vi "CompileParseRFPulse.vi"(0 "String":string) -> (2 "Array":variant[](array[variant]))   [LabVIEW 2019]
panel:
  out "output cluster":T1
  in  "Channel cluster":T2(array[cluster])
  in  "Timing cluster":T3
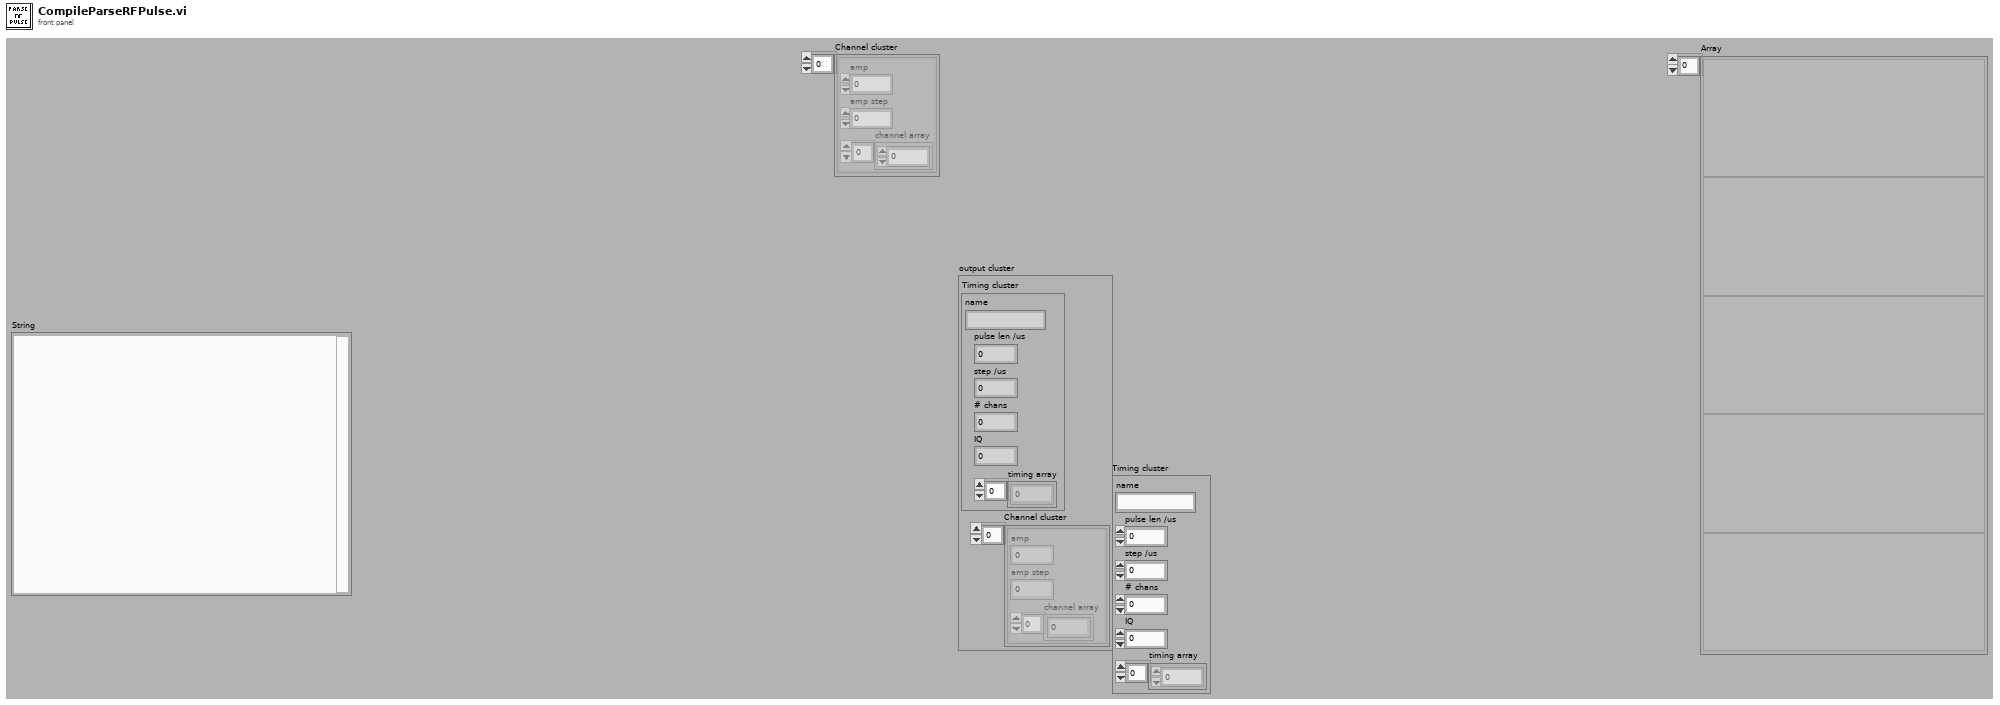
[diagram p1: front panel]
types:
  T1 = cluster{"Timing cluster":cluster{"name":string, "pulse len /us":dbl, "step /us":dbl, "# chans":i32, "IQ":i32, "timing array":dbl[]}, "Channel cluster":cluster{"amp":dbl, "amp step":dbl, "channel array":dbl[]}[]}
  T2 = cluster{"amp":dbl, "amp step":dbl, "channel array":dbl[]}[]
  T3 = cluster{"name":string, "pulse len /us":dbl, "step /us":dbl, "# chans":i32, "IQ":i32, "timing array":dbl[]}
  T4 = cluster{"Timing cluster 2":cluster{"name":string, "pulse len /us":dbl, "step /us":dbl, "# chans":i32, "IQ":i32, "timing array":dbl[]}, "Channel cluster 2":cluster{"amp":dbl, "amp step":dbl, "channel array":dbl[]}[]}
  T5 = cluster{"amp":dbl, "amp step":dbl, "array type (2D Dbl)":dbl[]}
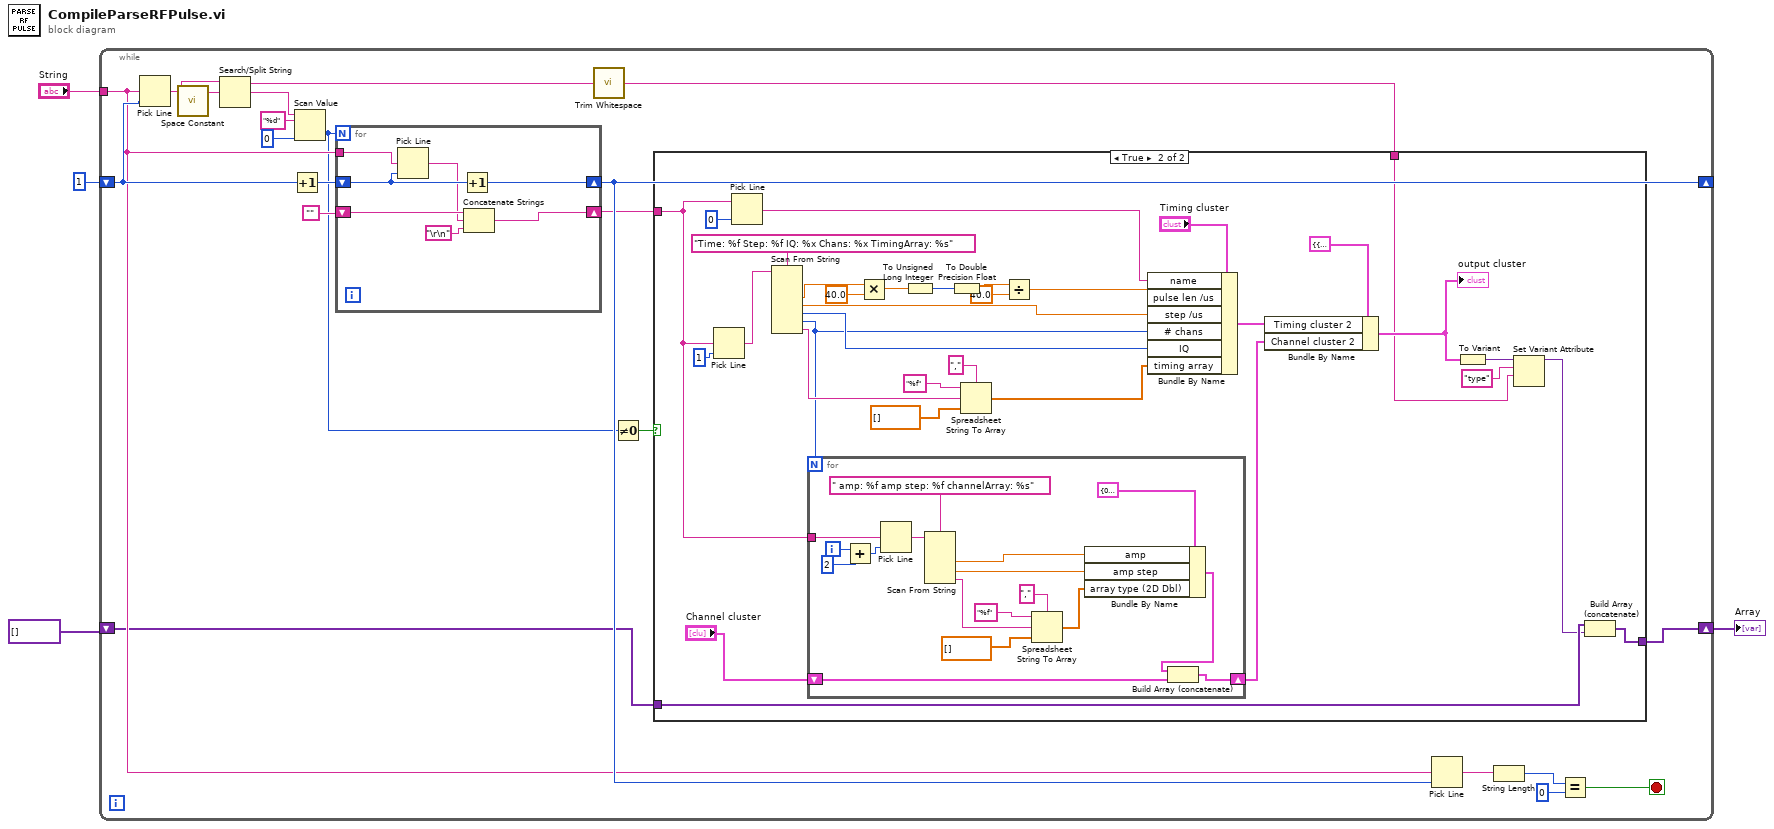
[diagram p0: block diagram]
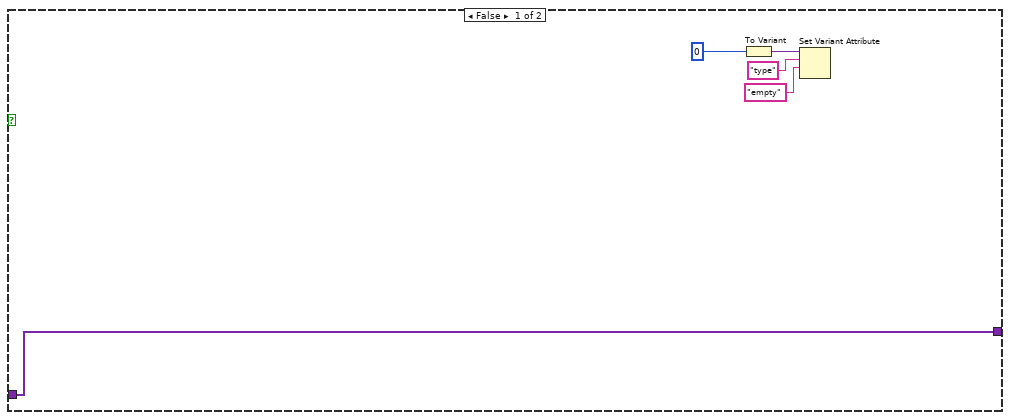
[diagram p2: hidden frame]
diagram:
  n1 = while {
    tunnel: "String" -> [w12]
    shift-right: [w13] -> _
    shift-left: 1 -> [w19]
    shift-right: [w6] -> w1
    shift-left: variant[] [] -> [w5]
    stop <- w14 stop-if-true
    n2 = Pick Line(multi-line string=w12, line index=w19) -> (output string=w25:string)  [unwired: 1 in]
    n3 = call <vilib>:"Space Constant.vi"() -> ("String"=w24:string)
    n4 = Search/Split String(string=w25, search string/char (-)=w24) -> (substring before match=w23:string, match + rest of string=w22:string)  [unwired: 1 in, 1 out]
    n5 = Increment(x=w19) -> (x+1=w18:i32)
    n6 = Scan Value(string=w22, format string="%d", default (0 dbl)=0) -> (value=w7:i32)  [unwired: 1 out]
    n7 = for {
      N: w7 -> [_]
      tunnel: w12 -> [w85]
      shift-right: [w87] -> w13
      shift-left: w18 -> [w86]
      shift-right: [w81] -> w11
      shift-left: "" -> [w84]
      n8 = Pick Line(multi-line string=w85, line index=w86) -> (output string=w83:string)  [unwired: 1 in]
      n9 = Increment(x=w86) -> (x+1=w87:i32)
      n10 = Concatenate Strings(w84, w83, "\r\n") -> (w81:string)
    }
    n11 = call <vilib>:"Trim Whitespace.vi"("string"=w23) -> ("trimmed string"=w9:string)  [unwired: 1 in]
    n12 = Not Equal To 0?(x=w7) -> (x != 0?=w8:bool)
    n13 = case shown="True" w8 {
      tunnel: w11 -> [_ w63]
      tunnel: w9 -> [_ w42]
      tunnel: [w26 w40] -> w6
      tunnel: w5 -> [w26 w39]
      frame False {
        n14 = To Variant(anything=0) -> (Variant=w29:variant)
        n15 = Set Variant Attribute(Variant=w29, name="type", value="empty" ("name")) -> ()  [unwired: 1 in, 3 out]
      }
      frame True {
        n16 = Pick Line(multi-line string=w63, line index=1) -> (output string=w62:string)  [unwired: 1 in]
        n17 = Pick Line(multi-line string=w63, line index=0) -> (output string=w49:string)  [unwired: 1 in]
        n18 = Scan From String(format string="Time: %f Step: %f IQ: %x Chans: %x TimingArray: %s", input string=w62) -> (output 1=w37:dbl, output 2=w61:dbl, output 3=w52:u32, output 4=w51:u32, output 5=w54:string)  [unwired: 7 in, 3 out]
        n19 = for {
          N: w51 -> [_]
          shift-right: [w68] -> w46
          shift-left: "Channel cluster" -> [w69]
          tunnel: w63 -> [w79]
          i -> [w78]
          n20 = Add(x=w78, y=2) -> (x+y=w77:i32)
          n21 = Pick Line(multi-line string=w79, line index=w77) -> (output string=w75:string)  [unwired: 1 in]
          n22 = Scan From String(format string=" amp: %f amp step: %f channelArray: %s", input string=w75) -> (output 1=w64:dbl, output 2=w65:dbl, output 3=w71:string)  [unwired: 5 in, 3 out]
          n23 = Spreadsheet String To Array(delimiter (Tab)=",", format string="%f", spreadsheet string=w71, array type (2D Dbl)=dbl[] []) -> (array=w66:dbl[])
          n24 = Bundle By Name(cluster=T5 {"amp"=0.0, "amp step"=0.0, "array type (2D Dbl)"=[]} ("freq cluster"), "amp"=w64, "amp step"=w65, "array type (2D Dbl)"=w66) -> (w67:T5)
          n25 = Build Array (concatenate)(w67, w69) -> (w68:T2)
        }
        n26 = Multiply(x=w37, y=40.0) -> (x*y=w35:dbl)
        n27 = To Unsigned Long Integer(number=w35) -> (unsigned 32bit integer=w34:u32)
        n28 = To Double Precision Float(number=w34) -> (double precision float=w33:dbl)
        n29 = Spreadsheet String To Array(delimiter (Tab)=",", format string="%f", spreadsheet string=w54, array type (2D Dbl)=dbl[] []) -> (array=w50:dbl[])
        n30 = Divide(x=w33, y=40.0) -> (x/y=w31:dbl)
        n31 = Bundle By Name(cluster="Timing cluster", "name"=w49, "pulse len /us"=w31, "step /us"=w61, "# chans"=w51, "IQ"=w52, "timing array"=w50) -> (w47:T3)
        n32 = Bundle By Name(cluster=T4 {"Timing cluster 2"={"name"="", "pulse len /us"=0.0, "step /us"=0.0, "# chans"=0, "IQ"=0, "timing array"=[]}, "Channel cluster 2"=[]} ("RF pulse cluster"), "Timing cluster 2"=w47, "Channel cluster 2"=w46) -> (w45:T4)
        "output cluster" <- w45
        n33 = To Variant(anything=w45) -> (Variant=w44:variant)
        n34 = Set Variant Attribute(Variant=w44, name="type", value=w42) -> (Variant out=w38:variant)  [unwired: 1 in, 2 out]
        n35 = Build Array (concatenate)(w39, w38) -> (w40:variant[])
      }
    }
    n36 = Pick Line(multi-line string=w12, line index=w13) -> (output string=w17:string)  [unwired: 1 in]
    n37 = String Length(string=w17) -> (length=w16:i32)
    n38 = Equal?(x=w16, y=0) -> (x = y?=w14:bool)
  }
  "Array" <- w1
